vi "TCP Test Client.vi"() -> ()   [LabVIEW 2020]
panel:
  out "error":errorcluster
  in  "IP Address":string="localhost"
  in  "Port":i32=4900
  in  "Command":string
  in  "Send":bool
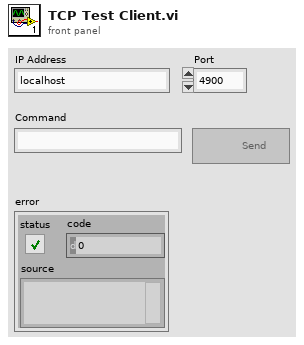
[diagram p1: front panel]
types:
  T1 = enum8{"Enabled", "Disabled", "Disabled and Grayed Out"}
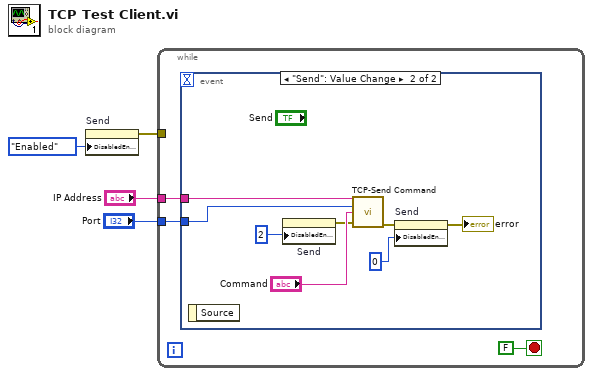
[diagram p0: block diagram]
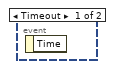
[diagram p2: hidden frame]
diagram:
  n1 = property on="Send" class="Bool"("DisabledEnum"=T1."Enabled" ("Disabled")) -> (error out=w2:errorcluster)  [unwired: 2 in, 1 out]
  n2 = while {
    tunnel: "IP Address" -> [w7]
    tunnel: "Port" -> [w6]
    tunnel: w2 -> [_]
    stop <- FALSE stop-if-true
    n3 = event shown="[1] \"Send\": Value Change" {
      selector: _ -> [_ _]
      dyn-events: _ -> [_ _]
      timeout: _ -> [_ _]
      tunnel: w7 -> [_ w15]
      tunnel: w6 -> [_ w14]
      event Timeout {
        n4 = event-data() -> ()  [unwired: 1 in, 1 out]
      }
      event "Send": Value Change {
        n5 = event-data() -> ()  [unwired: 1 in, 1 out]
        n6 = property on="Send" class="Bool"("DisabledEnum"=2) -> (error out=w12:errorcluster)  [unwired: 2 in, 1 out]
        n7 = call "TCP-Send Command.vi"("PXI Address"=w15, "Port"=w14, "Command"="Command", "error in (no error)"=w12) -> ("error out"=w10:errorcluster)  [unwired: 11 in]
        n8 = property on="Send" class="Bool"(error in=w10, "DisabledEnum"=0) -> (error out=→"error":errorcluster)  [unwired: 1 in, 1 out]
      }
    }
  }
